vi "PXDAC4800_ConnectToDeviceXD48.vi"(0 "brdNum":u32=1) -> (1 "Handle Out":i32, 2 "Status":i32)   [LabVIEW 2016]
uses:
  PXDAC4800.dll
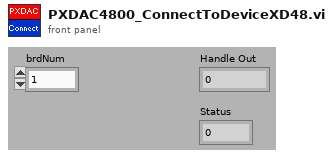
[diagram p1: front panel]
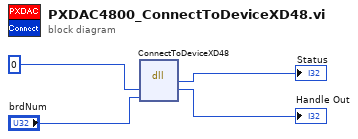
[diagram p0: block diagram]
diagram:
  n1 = dll-call lib="PXDAC4800.dll" fn="ConnectToDeviceXD48"("Handle"=0, "brdNum"="brdNum") -> (→"Status":i32, "Handle"=→"Handle Out":i32)  [unwired: 4 in, 2 out]
